vi "Test Process In Process Loop True when Uninitialized.vi"(8 "error in (no error)":errorcluster, 11 "Process Test In":refnum<class "Process Dev Test.lvclass">) -> (0 "error out":errorcluster, 3 "Process Test Out":refnum<class "Process Dev Test.lvclass">)   [LabVIEW 2020, in "Process Dev Test.lvclass"]
uses:
  Process Dev Test.lvclass
  Process Dev Test.lvclass/Process Dev Test.ctl
  source/Framework/Process/Process.lvclass
  <vilib>/Astemes/LUnit/Test Case.lvclass
  C:/git/astemes-triarc-framework/source/Framework Test Suite/Base Class Test/Base Test.lvclass
  C:/Program Files (x86)/National Instruments/LabVIEW 2020/vi.lib/Astemes/LUnit/Test Case.lvclass
  C:/Program Files (x86)/National Instruments/LabVIEW 2020/vi.lib/Astemes/LUnit/LUnit Runnable.lvclass
  C:/git/astemes-triarc-framework/tests/Process Development Test/Process Test/Process Dev Test.lvclass
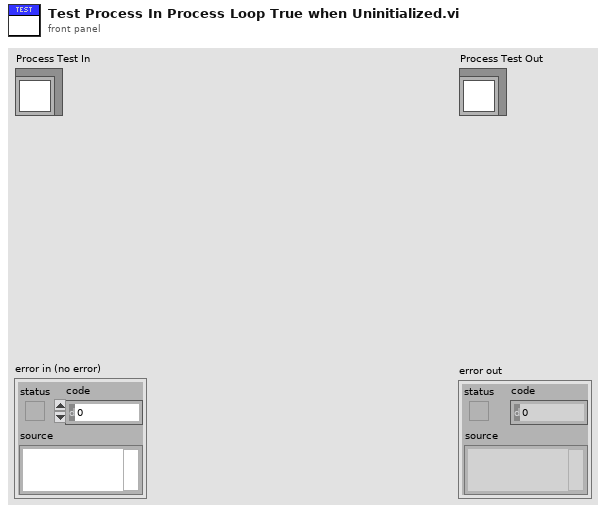
[diagram p1: front panel]
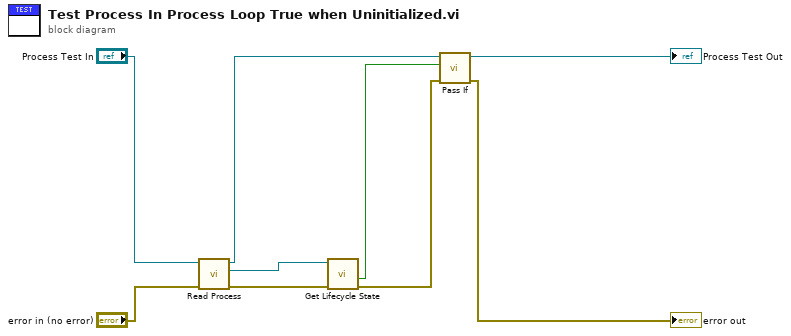
[diagram p0: block diagram]
diagram:
  n1 = call "Read Process.vi"("error in (no error)"="error in (no error)", "Process Test in"="Process Test In") -> ("error out"=w4:errorcluster, "Process.lvclass"=w5:refnum<class "Process.lvclass">, "Process Test out"=w2:refnum<class "Process Dev Test.lvclass">)  [unwired: 7 in]
  n2 = call "Get Lifecycle State.vi"("error in (no error)"=w4, "Process In"=w5) -> ("error out"=w8:errorcluster, "In Process Loop?"=w1:bool)  [unwired: 6 in, 2 out]
  n3 = call <vilib>:"Pass If.vi"("error in (no error)"=w8, "Pass?"=w1, "LUnit Test Case In"=w2) -> ("error out"=→"error out":errorcluster, "LUnit Test Case Out"=→"Process Test Out":refnum<class "Process Dev Test.lvclass">)  [unwired: 7 in]
